vi "Victory Dialog.vi"(9 "Pane Color":u32, 10 "Victory Phrase":string) -> ()   [LabVIEW 2015, in "SB SubVIs.lvlib"]
uses:
  SB SubVIs.lvlib
  Endigit Library/Endigit.lvlib
panel:
  in  "Finished":bool
  out "Victory Phrase out":string
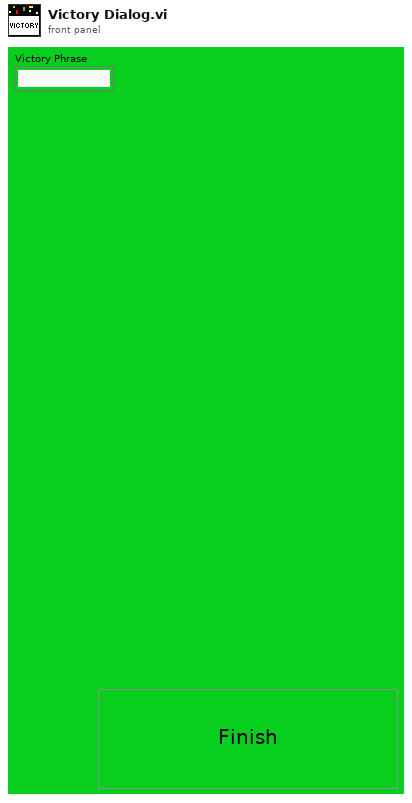
[diagram p1: front panel]
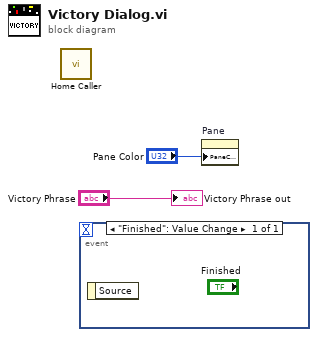
[diagram p0: block diagram]
diagram:
  n1 = call "Home Caller.vi"() -> ()  [unwired: 11 in]
  n2 = event shown="[0] \"Finished\": Value Change" {
    selector: _ -> [_]
    dyn-events: _ -> [_]
    timeout: _ -> [_]
    event "Finished": Value Change {
      n3 = event-data() -> ()  [unwired: 1 in, 1 out]
    }
  }
  n4 = property on="Pane" class="Pane"("PaneColor"="Pane Color") -> ()  [unwired: 2 in, 2 out]
  "Victory Phrase out" <- "Victory Phrase"
